vi "Show Connections.vi"(8 "error in (no error)":errorcluster, 11 "Server UI in":refnum<class "Server UI.lvclass">) -> (0 "error out":errorcluster, 3 "Server UI out":refnum<class "Server UI.lvclass">)   [LabVIEW 2026, in "Server UI.lvlib" / "Server UI.lvclass"]
uses:
  Server UI.lvclass
  C:/Program Files/National Instruments/LabVIEW 2026/vi.lib/ActorFramework/Actor/Actor.lvclass
  C:/Users/E2013170/Documents/GitHub/Measurement-Utility-Reference/source/framework/User Interface/UI.lvclass
  Server UI.lvclass/Server UI.ctl
  <vilib>/ActorFramework/Actor/Actor.lvclass/Actor.ctl
  framework/User Interface/UI.lvclass/UI.ctl
  <vilib>/ActorFramework/Message Enqueuer/Message Enqueuer.lvclass/Message Enqueuer.ctl
  Read Connection Showing.vi
  Read Start Server.vi
  Write Connection Showing.vi
  <vilib>/ActorFramework/Message Enqueuer/Enqueue.vi
  Controller/Messages/Launch Listener Msg/Launch Listener Msg.lvclass
  C:/Program Files/National Instruments/LabVIEW 2026/vi.lib/ActorFramework/Message/Message.lvclass
  Controller/Messages/Stop Listener Msg/Stop Listener Msg.lvclass
  <vilib>/ActorFramework/Message Priority Queue/Priority Enqueue.vi
  framework/User Interface/UI.lvclass
  <vilib>/ActorFramework/Actor/Actor.lvclass
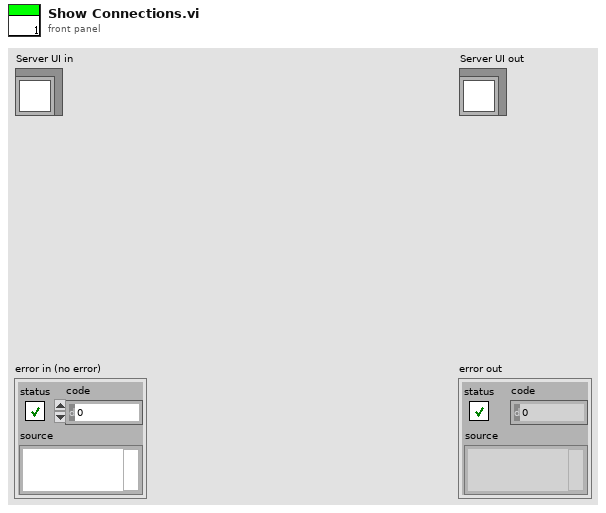
[diagram p1: front panel]
types:
  T1 = typedef "LVRectTypeDef.ctl" = cluster{"Left":i16, "Top":i16, "Right":i16, "Bottom":i16}
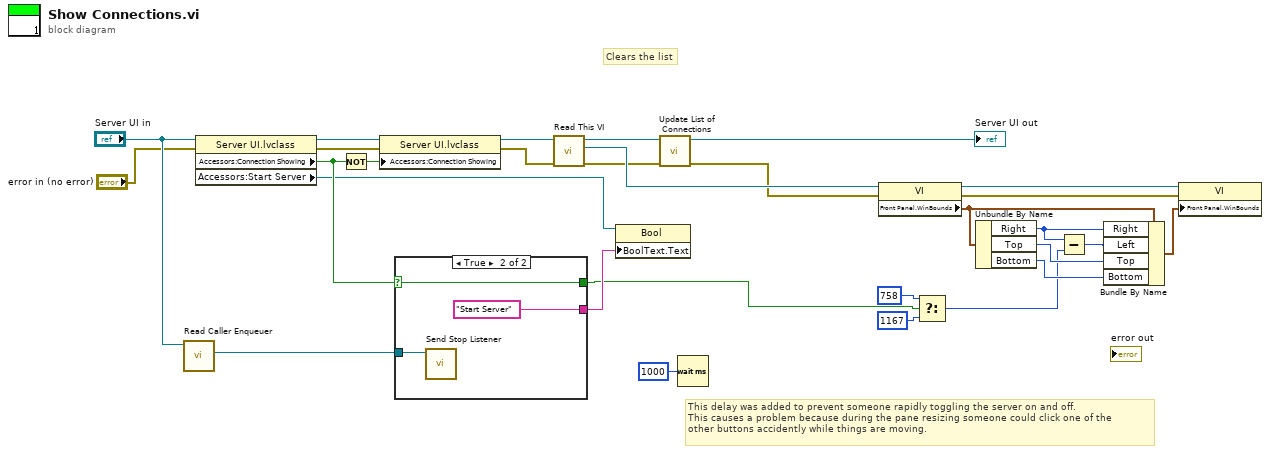
[diagram p0: block diagram]
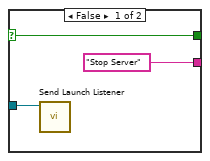
[diagram p2: hidden frame]
diagram:
  # "Clears the list"
  # "This delay was added to prevent someone rapidly toggling the server on and off.\nThis causes a problem because during the pane resizing someone could click one of the \nother buttons accidently while things are moving."
  n1 = call <vilib>:"Read Caller Enqueuer.vi"("Actor"="Server UI in") -> ("Caller Enqueuer"=w14:refnum<class "Message Enqueuer.lvclass">)  [unwired: 10 in]
  n2 = property class="Server UI.lvclass"(reference="Server UI in", error in="error in (no error)") -> (reference out=w19:refnum<class "Server UI.lvclass">, error out=w5:errorcluster, "Accessors:Connection Showing"=w16:bool, "Accessors:Start Server"=w11:refnum<vi>)
  n3 = Not(x=w16) -> (.not. x?=w17:bool)
  n4 = property class="Server UI.lvclass"(reference=w19, error in=w5, "Accessors:Connection Showing"=w17) -> (reference out=w18:refnum<class "Server UI.lvclass">, error out=w4:errorcluster)
  n5 = case shown="True" w16 {
    selector: w16 -> [w30 w33]
    tunnel: w14 -> [w32 w35]
    tunnel: ["Stop Server" ("Boolean Text.Text") "Start Server" ("Boolean Text.Text")] -> w12
    tunnel: [w30 w33] -> w3
    frame False {
      n6 = call "Send Launch Listener.vi"("Message Enqueuer"=w32) -> ()  [unwired: 9 in, 2 out]
    }
    frame True {
      n7 = call "Send Stop Listener.vi"("Message Enqueuer"=w35) -> ()  [unwired: 9 in, 2 out]
    }
  }
  n8 = call "Read This VI.vi"("error in (no error)"=w4, "UI in"=w18) -> ("error out"=w2:errorcluster, "This VI"=w8:refnum<vi>, "UI out"=w10:refnum<class "Server UI.lvclass">)  [unwired: 7 in]
  n9 = property class="Bool"(reference=w11, "BoolText.Text"=w12) -> ()  [unwired: 1 in, 2 out]
  n10 = call "Update List of Connections.vi"("error in (no error)"=w2, "Server UI in"=w10) -> ("error out"=w1:errorcluster, "Server UI out"=→"Server UI out":refnum<class "Server UI.lvclass">)  [unwired: 8 in]
  n11 = Wait (ms)(milliseconds to wait=u32 1000) -> ()  [unwired: 1 out]
  n12 = property class="VI"(reference=w8, error in=w1) -> (reference out=w29:refnum<vi>, error out=w25:errorcluster, "Front Panel.WinBounds"=w28:T1)
  n13 = Select(t=i16 758 ("y"), s=w3, f=i16 1167 ("y")) -> (s? t:f=w21:i16)
  n14 = Unbundle By Name(w28) -> ("Right"=w13:i16, "Top"=w23:i16, "Bottom"=w24:i16)
  n15 = Subtract(x=w13, y=w21) -> (x-y=w26:i16)
  n16 = Bundle By Name(cluster=w28, "Right"=w13, "Left"=w26, "Top"=w23, "Bottom"=w24) -> (w27:T1)
  n17 = property class="VI"(reference=w29, error in=w25, "Front Panel.WinBounds"=w27) -> ()  [unwired: 2 out]
